vi "Pneumatics.vi"(11 "Pneumatic Mode":T1(ring)) -> ()   [LabVIEW 2013]
uses:
  <vilib>/Rock Robotics/WPI/Relay/WPI_RelayValue.ctl
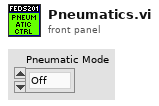
[diagram p1: front panel]
types:
  T1 = enum16{"Off", "Charge 1", "Charge 2", "Charge 3", "Shoot", "Lock", "Arm Up", "Arm Down", "Kicker"}
  T2 = typedef "WPI_RelayValue.ctl" = enum16{"Off", "On", "Forward", "Reverse"}
  T3 = typedef "WPI_RelayDevRef.ctl" = cluster{"DevStatus":errorcluster, "Relay Channel":T4, "Digital Module":T5, "Relay Direction":T6}
  T4 = typedef "FPGA_DIORelayChannel.ctl" = enum8{"Relay 1", "Relay 2", "Relay 3", "Relay 4", "Relay 5", "Relay 6", "Relay 7", "Relay 8", "Invalid"}
  T5 = typedef "FPGA_TypedefDigitalModule.ctl" = enum16{"Digital Module 1", "Digital Module 2"}
  T6 = typedef "WPI_RelayDirection.ctl" = enum16{"Both directions", "Forward only", "Reverse only"}
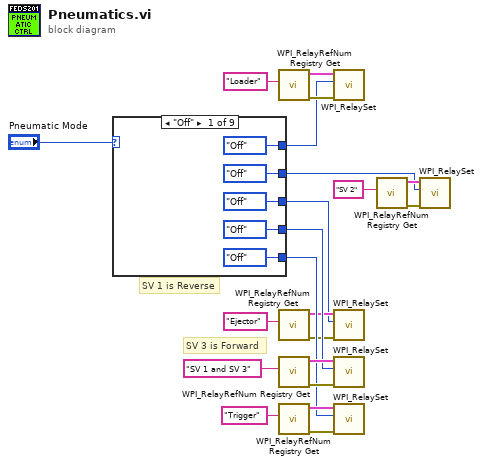
[diagram p0: block diagram]
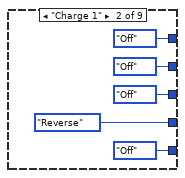
[diagram p2: hidden frame]
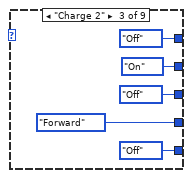
[diagram p3: hidden frame]
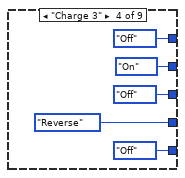
[diagram p4: hidden frame]
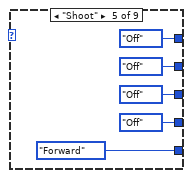
[diagram p5: hidden frame]
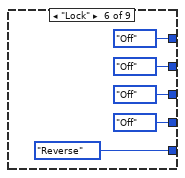
[diagram p6: hidden frame]
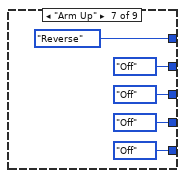
[diagram p7: hidden frame]
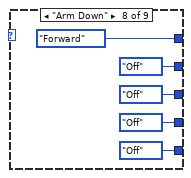
[diagram p8: hidden frame]
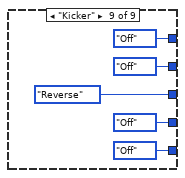
[diagram p9: hidden frame]
diagram:
  # "SV 3 is Forward"
  # "SV 1 is Reverse"
  n1 = case shown="\"Off\"" "Pneumatic Mode" {
    tunnel: [WPI_RelayValue."Off" ("RelayValue") WPI_RelayValue."Reverse" ("RelayValue") WPI_RelayValue."Forward" ("RelayValue") WPI_RelayValue."Reverse" ("RelayValue") WPI_RelayValue."Off" ("RelayValue") WPI_RelayValue."Off" ("RelayValue") WPI_RelayValue."Off" ("RelayValue") WPI_RelayValue."Off" ("RelayValue") WPI_RelayValue."Off" ("RelayValue")] -> w14
    tunnel: [WPI_RelayValue."Off" ("RelayValue") WPI_RelayValue."Off" ("RelayValue") WPI_RelayValue."On" ("RelayValue") WPI_RelayValue."On" ("RelayValue") WPI_RelayValue."Off" ("RelayValue") WPI_RelayValue."Off" ("RelayValue") WPI_RelayValue."Off" ("RelayValue") WPI_RelayValue."Off" ("RelayValue") WPI_RelayValue."Off" ("RelayValue")] -> w13
    tunnel: [WPI_RelayValue."Off" ("RelayValue") WPI_RelayValue."Off" ("RelayValue") WPI_RelayValue."Off" ("RelayValue") WPI_RelayValue."Off" ("RelayValue") WPI_RelayValue."Forward" ("RelayValue") WPI_RelayValue."Reverse" ("RelayValue") WPI_RelayValue."Off" ("RelayValue") WPI_RelayValue."Off" ("RelayValue") WPI_RelayValue."Off" ("RelayValue")] -> w10
    tunnel: [WPI_RelayValue."Off" ("RelayValue") WPI_RelayValue."Off" ("RelayValue") WPI_RelayValue."Off" ("RelayValue") WPI_RelayValue."Off" ("RelayValue") WPI_RelayValue."Off" ("RelayValue") WPI_RelayValue."Off" ("RelayValue") WPI_RelayValue."Reverse" ("RelayValue") WPI_RelayValue."Forward" ("RelayValue") WPI_RelayValue."Off" ("RelayValue")] -> w3
    tunnel: [WPI_RelayValue."Off" ("RelayValue") WPI_RelayValue."Off" ("RelayValue") WPI_RelayValue."Off" ("RelayValue") WPI_RelayValue."Off" ("RelayValue") WPI_RelayValue."Off" ("RelayValue") WPI_RelayValue."Off" ("RelayValue") WPI_RelayValue."Off" ("RelayValue") WPI_RelayValue."Off" ("RelayValue") WPI_RelayValue."Reverse" ("RelayValue")] -> w2
    frame "Off" {
    }
    frame "Charge 1" {
    }
    frame "Charge 2" {
    }
    frame "Charge 3" {
    }
    frame "Shoot" {
    }
    frame "Lock" {
    }
    frame "Arm Up" {
    }
    frame "Arm Down" {
    }
    frame "Kicker" {
    }
  }
  n2 = call <vilib>:"WPI_RelayRefNum Registry Get.vi"("refnum name"="Loader") -> ("error out"=w7:errorcluster, "RelayDevRef"=w8:T3)  [unwired: 9 in]
  n3 = call <vilib>:"WPI_RelayRefNum Registry Get.vi"("refnum name"="Ejector") -> ("error out"=w6:errorcluster, "RelayDevRef"=w4:T3)  [unwired: 9 in]
  n4 = call <vilib>:"WPI_RelayRefNum Registry Get.vi"("refnum name"="SV 1 and SV 3") -> ("error out"=w21:errorcluster, "RelayDevRef"=w17:T3)  [unwired: 9 in]
  n5 = call <vilib>:"WPI_RelayRefNum Registry Get.vi"("refnum name"="Trigger") -> ("error out"=w1:errorcluster, "RelayDevRef"=w12:T3)  [unwired: 9 in]
  n6 = call <vilib>:"WPI_RelaySet.vi"("error in (no error)"=w7, "RelayValue"=w3, "RelayDevRef"=w8) -> ()  [unwired: 7 in, 2 out]
  n7 = call <vilib>:"WPI_RelaySet.vi"("error in (no error)"=w6, "RelayValue"=w2, "RelayDevRef"=w4) -> ()  [unwired: 7 in, 2 out]
  n8 = call <vilib>:"WPI_RelaySet.vi"("error in (no error)"=w21, "RelayValue"=w14, "RelayDevRef"=w17) -> ()  [unwired: 7 in, 2 out]
  n9 = call <vilib>:"WPI_RelaySet.vi"("error in (no error)"=w1, "RelayValue"=w10, "RelayDevRef"=w12) -> ()  [unwired: 7 in, 2 out]
  n10 = call <vilib>:"WPI_RelayRefNum Registry Get.vi"("refnum name"="SV 2") -> ("error out"=w20:errorcluster, "RelayDevRef"=w19:T3)  [unwired: 9 in]
  n11 = call <vilib>:"WPI_RelaySet.vi"("error in (no error)"=w20, "RelayValue"=w13, "RelayDevRef"=w19) -> ()  [unwired: 7 in, 2 out]
